vi "tcp_客户端_接收.vi"(0 "IP地址":string="127.0.0.1" caption="对方公网访问地址", 1 "端口号":i32=6314, 2 "储存路径":path=path "D:/AA") -> ()   [LabVIEW 2016, in "自动更新.lvlib" / "TCP文件传输系统.lvlib" / "TCP接收文件.lvlib"]
panel:
  out "运行中":bool
  out "单包大小":i32
  in  "分一包（兆）":i64=40
  out "已收百分比":string
  out "帧数":i32
  out "帧号":i32
  out "生成新的保存路径":path
  out "需接收次数":i32
  out "文件名":string
  out "已收次数":i32
  out "error out":errorcluster
  out "当前步骤":T1(ring)
  out "错误输出":errorcluster
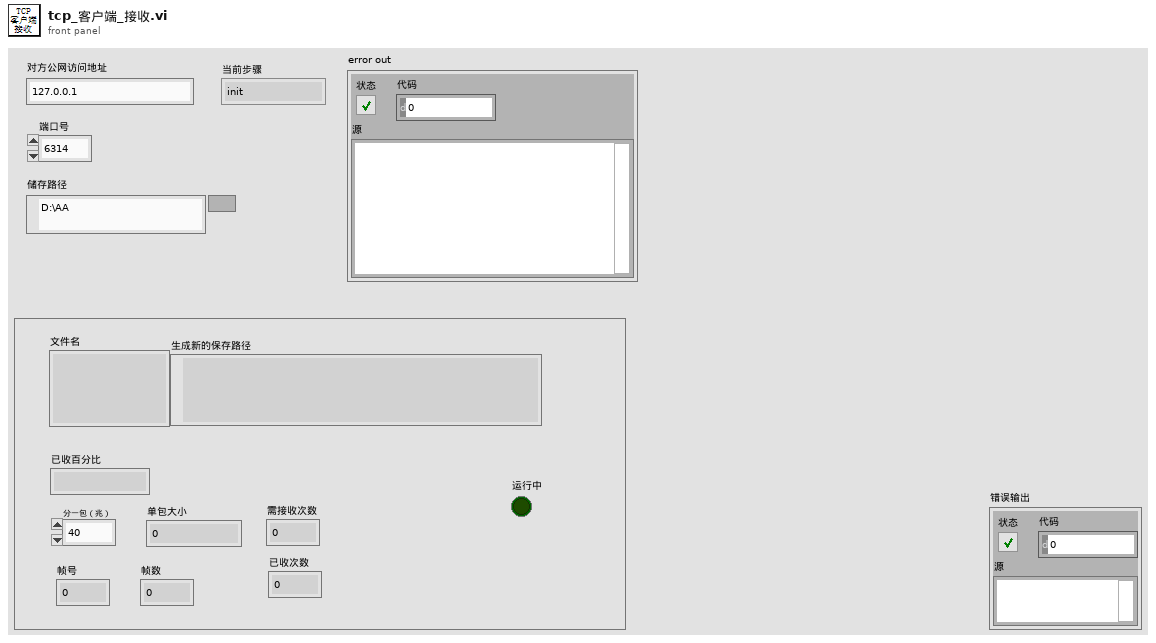
[diagram p1: front panel]
types:
  T1 = enum16{"init", "receivehead", "receivecontent", "receivesuccess", "over"}
  T2 = enum16{"open", "replace", "create", "open or create", "replace or create", "replace or create with confirmation"}
  T3 = cluster{"网络灯":bool, "接收中":bool, "已接收百分比":u8, "接收成功次数":dbl, "当前步骤":enum16{"init", "receivehead", "receivecontent", "receivesuccess", "over"}, "文件名":string, "error out":errorcluster}
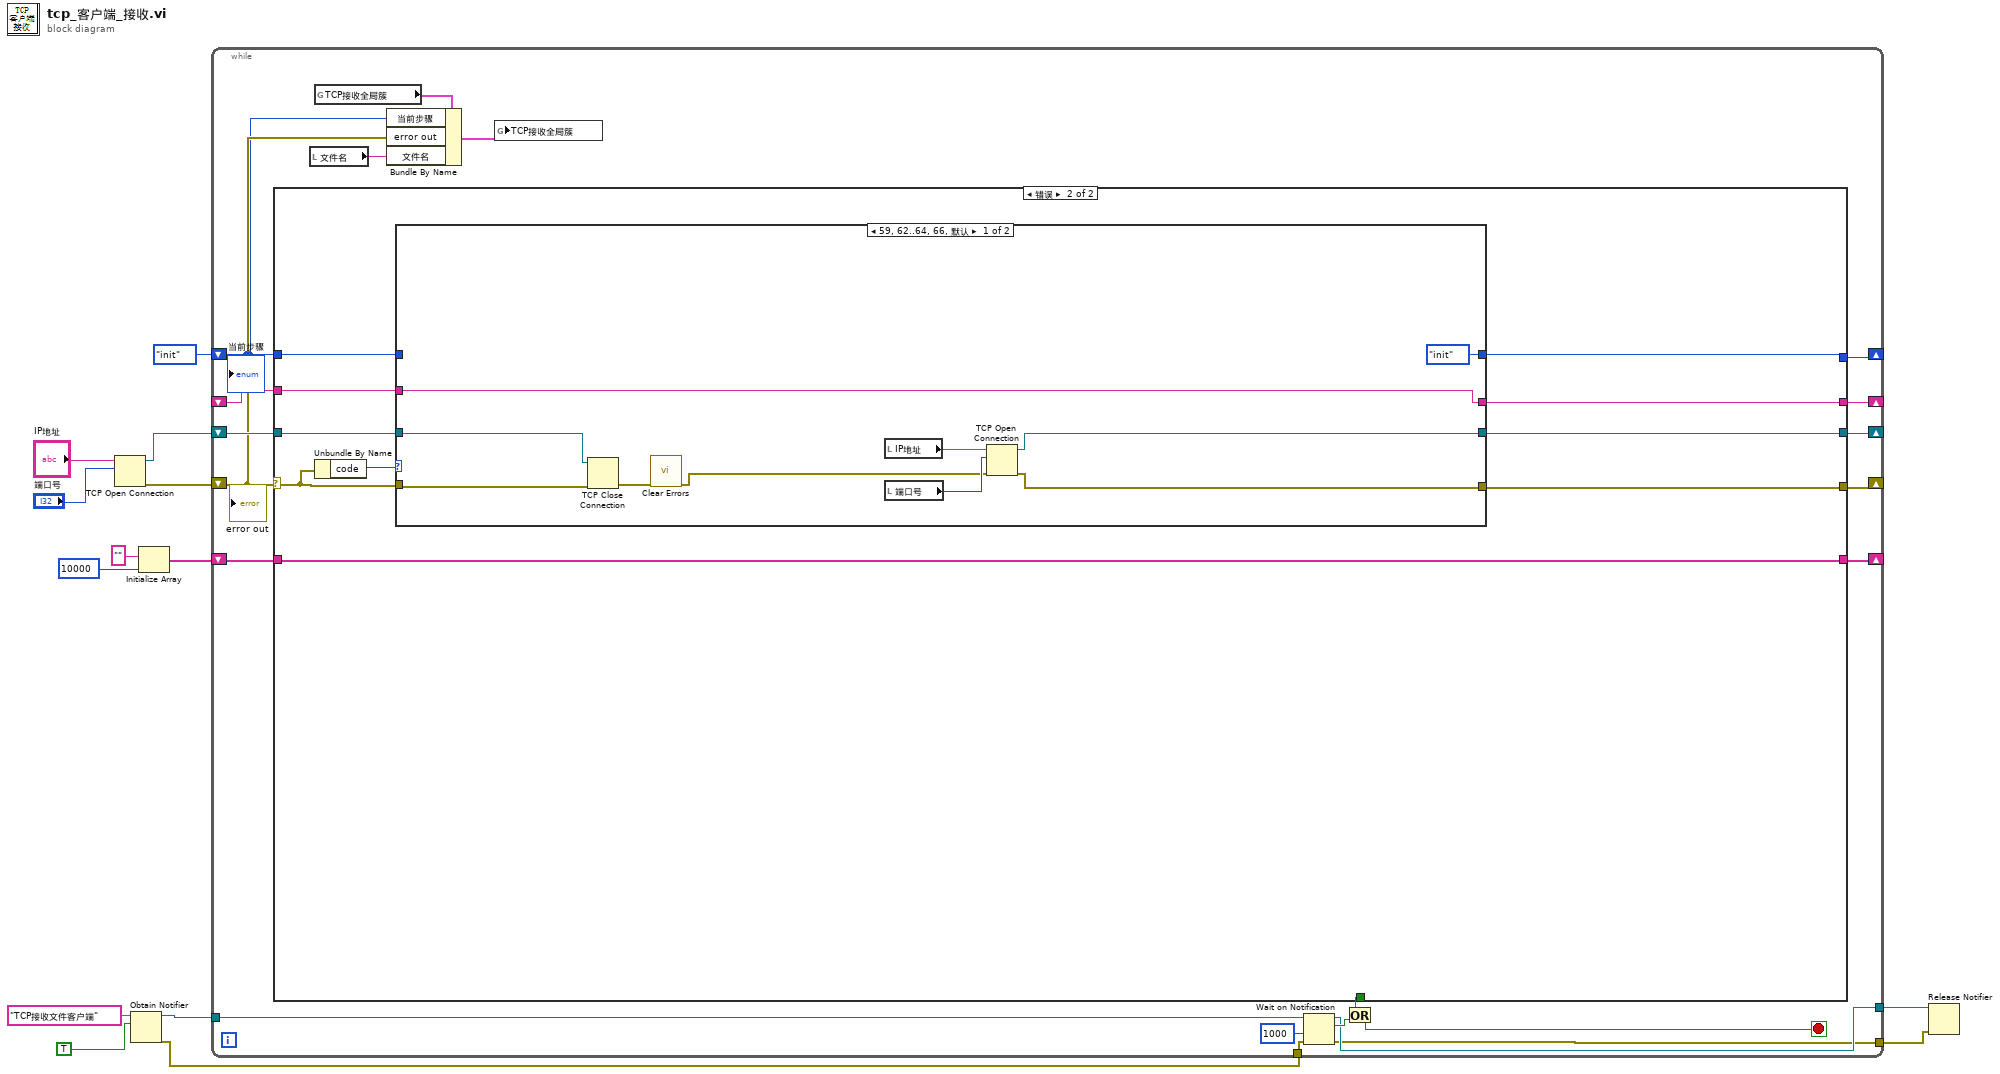
[diagram p0: block diagram]
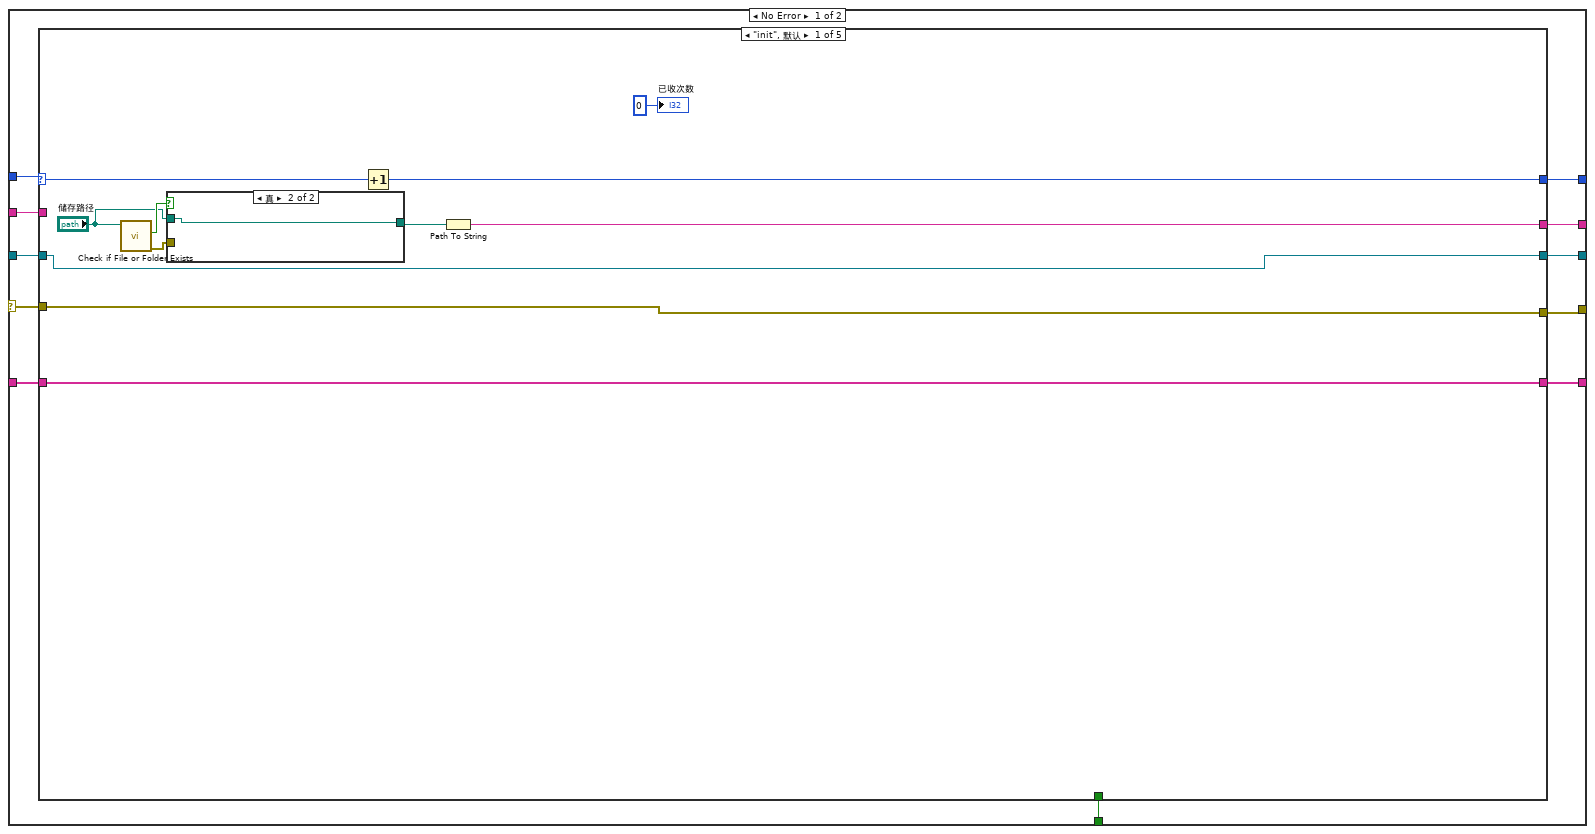
[diagram p2: hidden frame]
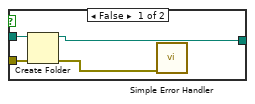
[diagram p3: hidden frame]
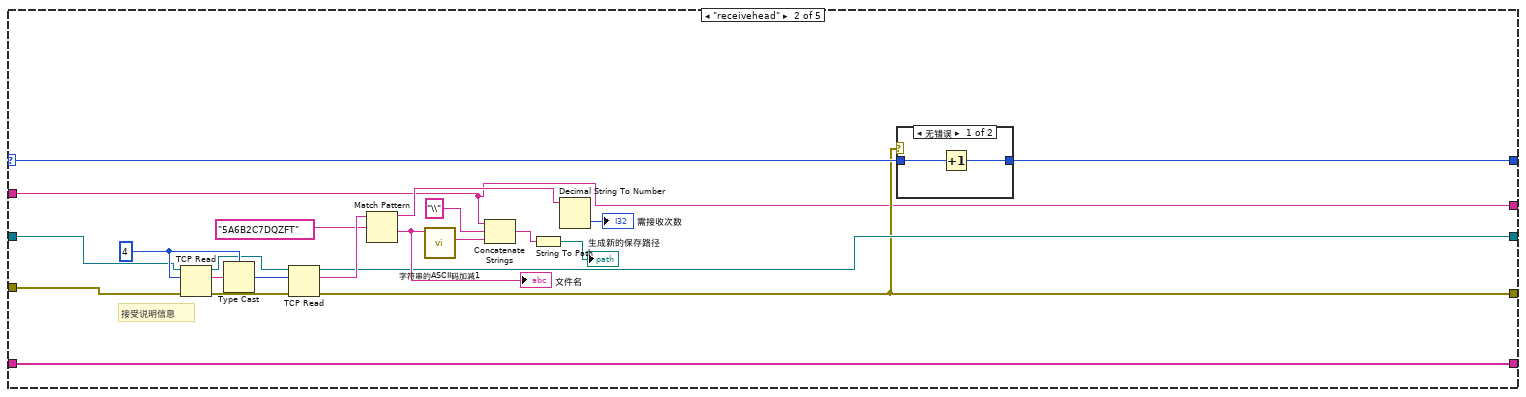
[diagram p4: hidden frame]
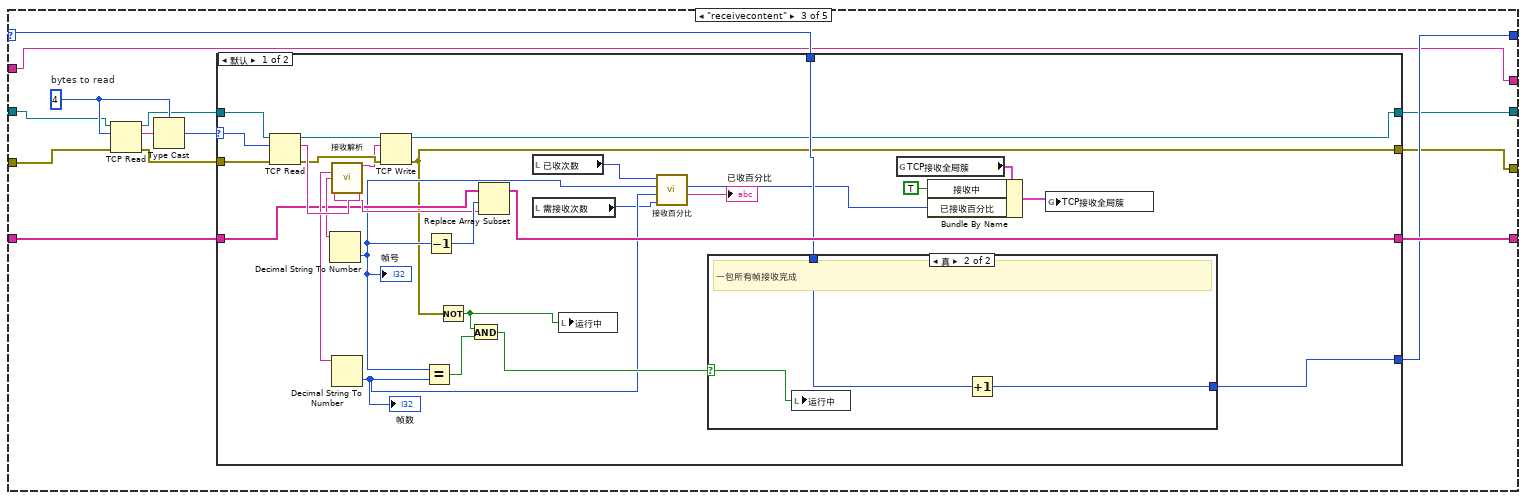
[diagram p6: hidden frame]
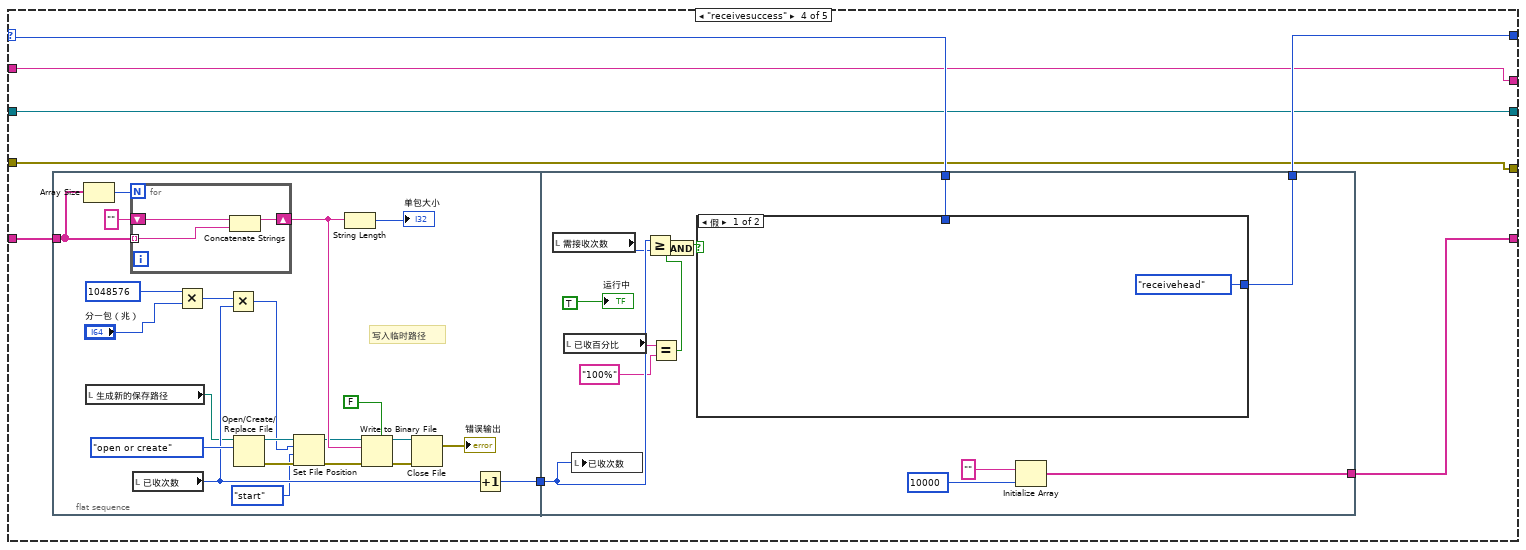
[diagram p9: hidden frame]
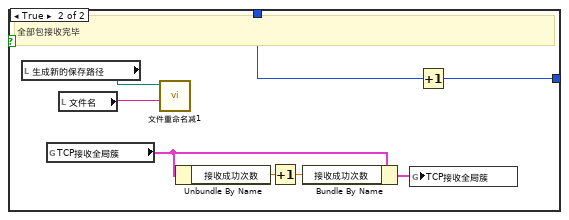
[diagram p10: hidden frame]
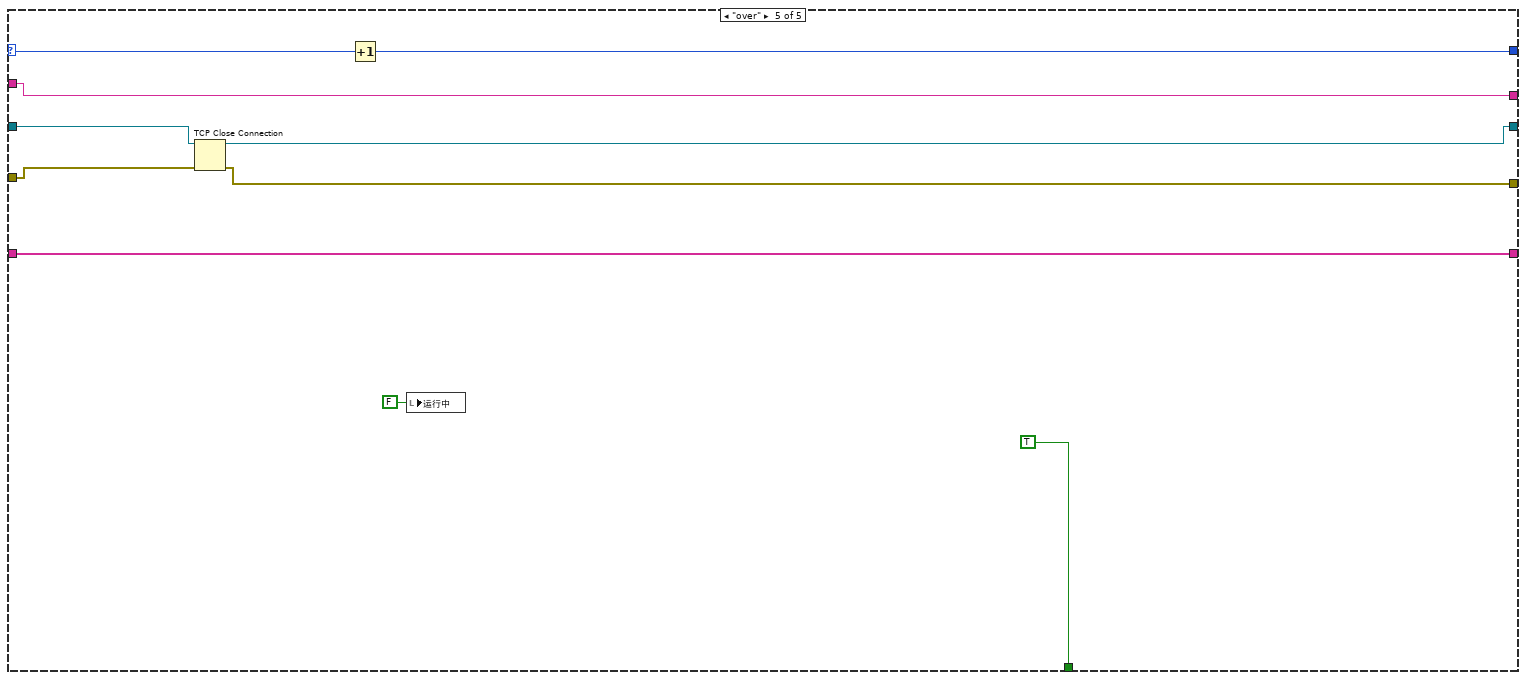
[diagram p11: hidden frame]
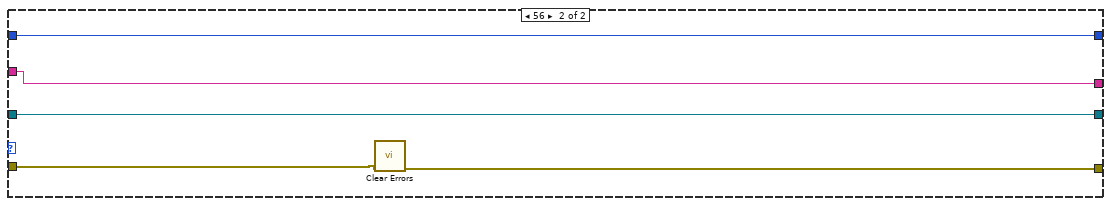
[diagram p12: hidden frame]
diagram:
  n1 = TCP Open Connection(address="IP地址", remote port or service name="端口号") -> (connection ID=w8:refnum<k5>, error out=w9:errorcluster)  [unwired: 3 in]
  n2 = Obtain Notifier(name (unnamed)="TCP接收文件客户端" ("名称（未命名）"), notification data type=TRUE) -> (notifier out=w6:refnum<notifier>, error out=w1:errorcluster)  [unwired: 2 in, 1 out]
  n3 = Initialize Array("", 10000 ("维数大小")) -> (w7:string[])
  n4 = while {
    shift-right: [w35] -> _
    shift-left: T1."init" -> [w16]
    shift-right: [w33] -> _
    shift-left: w9 -> [w17]
    shift-right: [w31] -> _
    shift-left: w8 -> [w32]
    shift-right: [w30] -> _
    shift-left: _ -> [w29]
    shift-right: [w27] -> _
    shift-left: w7 -> [w28]
    tunnel: w6 -> [w26]
    tunnel: [w22] -> w3
    tunnel: [w21] -> w2
    tunnel: w1 -> [w20]
    stop <- w25 stop-if-true
    n5 = case shown="错误" w17 {
      selector: w17 -> [w41 w212]
      tunnel: w16 -> [w46 w208]
      tunnel: [w45 w207] -> w35
      tunnel: [w44 _] -> w34
      tunnel: [w39 w211] -> w33
      tunnel: w32 -> [w42 w210]
      tunnel: [w38 w209] -> w31
      tunnel: [w43 w205] -> w30
      tunnel: w29 -> [w40 w206]
      tunnel: w28 -> [w37 w204]
      tunnel: [w36 w204] -> w27
      frame No Error {
        n6 = case shown="\"init\", 默认" w46 {
          selector: w46 -> [w57 w84 w92 w142 w203]
          tunnel: [w56 w83 w91 w143 w202] -> w45
          tunnel: [_ _ _ _ TRUE] -> w44
          tunnel: [w50 w64 w88 w139 w194] -> w43
          tunnel: w42 -> [w49 w75 w98 w140 w199]
          tunnel: w41 -> [w48 w74 w99 w141 w198]
          tunnel: w40 -> [_ w64 w88 w139 w194]
          tunnel: [w48 w65 w90 w141 w196] -> w39
          tunnel: [w49 w66 w89 w140 w197] -> w38
          tunnel: w37 -> [w47 w63 w96 w145 w195]
          tunnel: [w47 w63 w93 w144 w195] -> w36
          frame "init", Default {
            n7 = call <vilib>:"Check if File or Folder Exists.vi"("path"="储存路径") -> ("error out"=w53:errorcluster, "file or folder exists?"=w54:bool)  [unwired: 8 in, 1 out]
            n8 = case shown="真" w54 {
              tunnel: "储存路径" -> [w61 w62]
              tunnel: w53 -> [w60 _]
              tunnel: [w59 w62] -> w51
              frame False {
                n9 = Create Folder(path (use dialog)=w61, error in=w60) -> (created path=w59:path, error out=w58:errorcluster)  [unwired: 1 in, 1 out]
                n10 = call <vilib>:"Simple Error Handler.vi"("error in (no error)"=w58) -> ()  [unwired: 4 in, 5 out]
              }
              frame True {
              }
            }
            n11 = Increment(x=w57) -> (x+1=w56:T1)
            n12 = Path To String(path=w51) -> (string=w50:string)
            "已收次数" <- i64 0 ("已发次数")
          }
          frame "receivehead" {
            w82 = 4 ("读取的字节")
            # "接受说明信息"
            n13 = TCP Read(connection ID=w75, bytes to read=w82, error in (no error)=w74) -> (connection ID out=w78:refnum<k5>, data out=w81:string, error out=w79:errorcluster)  [unwired: 2 in]
            n14 = Type Cast(type=w82, x=w81) -> (*(type *) &x=w80:i32)
            n15 = TCP Read(connection ID=w78, bytes to read=w80, error in (no error)=w79) -> (connection ID out=w66:refnum<k5>, data out=w77:string, error out=w65:errorcluster)  [unwired: 2 in]
            n16 = Match Pattern(string=w77, regular expression="5A6B2C7DQZFT" ("正则表达式")) -> (before substring=w70:string, after substring=w73:string)  [unwired: 1 in, 2 out]
            "文件名" <- w73
            n17 = call "字符串的ASCII码加减1.vi"("原字符串"=w73) -> ("ASCII码"=w72:string)  [unwired: 10 in]
            n18 = Concatenate Strings(w64, "\\" ("字符串"), w72) -> (w67:string)
            n19 = String To Path(string=w67) -> (path=→"生成新的保存路径":path)
            n20 = Decimal String To Number(string=w70) -> (number=→"需接收次数":i32)  [unwired: 2 in, 1 out]
            n21 = case shown="无错误" w65 {
              tunnel: w84 -> [w86 w87]
              tunnel: [w85 w87] -> w83
              frame No Error {
                n22 = Increment(x=w86) -> (x+1=w85:T1)
              }
              frame Error {
              }
            }
          }
          frame "receivecontent" {
            w101 = 4  # bytes to read
            n23 = TCP Read(connection ID=w98, bytes to read=w101, error in (no error)=w99) -> (connection ID out=w95:refnum<k5>, data out=w100:string, error out=w94:errorcluster)  [unwired: 2 in]
            n24 = Type Cast(type=w101, x=w100) -> (*(type *) &x=w97:i32)
            n25 = case shown="默认" w97 {
              selector: w97 -> [w118 _]
              tunnel: w96 -> [w121 w137]
              tunnel: w95 -> [w120 w135]
              tunnel: w94 -> [w119 w136]
              tunnel: [w114 w137] -> w93
              tunnel: w92 -> [w112 w138]
              tunnel: [w111 w138] -> w91
              tunnel: [w110 w136] -> w90
              tunnel: [w109 w135] -> w89
              frame Default {
                n26 = TCP Read(connection ID=w120, bytes to read=w118, error in (no error)=w119) -> (connection ID out=w127:refnum<k5>, data out=w130:string, error out=w126:errorcluster)  [unwired: 2 in]
                n27 = call "接收解析.vi"("data in"=w130) -> ("重算CRC32"=w124:string, "帧数"=w125:string, "帧号"=w129:string, "帧内容"=w123:string)  [unwired: 3 in, 8 out]
                n28 = Decimal String To Number(string=w129) -> (number=w116:i32)  [unwired: 2 in, 1 out]
                "帧号" <- w116
                n29 = Decimal String To Number(string=w125) -> (number=w103:i32)  [unwired: 2 in, 1 out]
                "帧数" <- w103
                n30 = TCP Write(connection ID=w127, data in=w124, error in (no error)=w126) -> (connection ID out=w109:refnum<k5>, error out=w110:errorcluster)  [unwired: 1 in, 1 out]
                n31 = Equal?(x=w116, y=w103) -> (x = y?=w122:bool)
                n32 = Decrement(x=w116) -> (x-1=w128:i32)
                n33 = Not(x=w110) -> (.not. x?=w108:bool)
                n34 = And(x=w108, y=w122) -> (x .and. y?=w113:bool)
                n35 = Replace Array Subset(array=w121, new element=w123, index=w128) -> (w114:string[])
                n36 = local read "已收次数"() -> (w117:i32)
                n37 = local read "需接收次数"() -> (w102:i32)
                n38 = local write "运行中"(w108) -> ()
                n39 = call "接收百分比.vi"("需发送次数"=w102, "帧数"=w103, "帧号"=w116, "已收次数"=w117) -> (1:"已收百分比"=→"已收百分比":string, 2:"已收百分比"=w104:u8)  [unwired: 6 in]
                n40 = case shown="真" w113 {
                  selector: w113 -> [_ w132]
                  tunnel: w112 -> [w131 w134]
                  tunnel: [w131 w133] -> w111
                  frame False {
                    # "重复接收"
                  }
                  frame True {
                    # "一包所有帧接收完成"
                    n41 = local write "运行中"(w132) -> ()
                    n42 = Increment(x=w134) -> (x+1=w133:T1)
                  }
                }
                n43 = global read "全局变量1.vi" "TCP接收全局簇"() -> (w105:T3)
                n44 = Bundle By Name(cluster=w105, "接收中"=TRUE, "已接收百分比"=w104) -> (w106:T3)
                n45 = global write "全局变量1.vi" "TCP接收全局簇"(w106) -> ()
              }
              frame ..0 {
                # "content为空"
              }
            }
          }
          frame "receivesuccess" {
            n46 = flat-sequence {
              tunnel: w145 -> [w160]
              tunnel: [w168] -> w146
              tunnel: w146 -> [w178]
              tunnel: [w182] -> w144
              tunnel: w142 -> [w180]
              tunnel: [w179] -> w143
              frame #0 {
                # "写入临时路径"
                n47 = Array Size(array=w160) -> (size(s)=w161:i32)
                n48 = local read "生成新的保存路径"() -> (w147:path)
                n49 = for {
                  N: w161 -> [_]
                  shift-right: [w171] -> w159
                  shift-left: "" -> [w170]
                  tunnel: w160 -> [w169] mode=indexing
                  n50 = Concatenate Strings(w170, w169) -> (w171:string)
                }
                n51 = local read "已收次数"() -> (w153:i32)
                n52 = Multiply(x=i64 1048576, y="分一包（兆）") -> (x*y=w149:i64)
                n53 = Multiply(x=w149, y=w153) -> (x*y=w152:i64)
                n54 = Open/Create/Replace File(file path (use dialog)=w147, operation (0:open)=T2."open or create" ("操作(0:open)")) -> (refnum out=w156:refnum<file>, error out=w157:errorcluster)  [unwired: 4 in, 1 out]
                n55 = Set File Position(offset (in bytes) (0)=w152, refnum=w156, from (0:start)=enum16{"start", "end", "current"}."start" ("自（0:起始）"), error in=w157) -> (refnum out=w154:refnum<file>, error out=w155:errorcluster)
                n56 = String Length(string=w159) -> (length=→"单包大小":i32)
                n57 = Write to Binary File(file (use dialog)=w154, data=w159, error in=w155, 5:FALSE ("预置数组或字符串大小？(T)")) -> (refnum out=w166:refnum<file>, error out=w167:errorcluster)  [unwired: 2 in, 1 out]
                n58 = Close File(refnum=w166, error in=w167) -> (error out=→"错误输出":errorcluster)  [unwired: 1 out]
                n59 = Increment(x=w153) -> (x+1=w168:i32)
              }
              frame #1 {
                n60 = local read "需接收次数"() -> (w177:i32)
                n61 = local read "已收百分比"() -> (w175:string)
                n62 = local write "已收次数"(w178) -> ()
                n63 = Greater Or Equal?(x=w178, y=w177) -> (x >= y?=w176:bool)
                n64 = Equal?(x=w175, y="100%" ("已收百分比")) -> (x = y?=w172:bool)
                n65 = And(x=w176, y=w172) -> (x .and. y?=w173:bool)
                n66 = case shown="假" w173 {
                  tunnel: w180 -> [_ w187]
                  tunnel: [T1."receivehead" w186] -> w179
                  frame False {
                  }
                  frame True {
                    # "全部包接收完毕"
                    n67 = local read "生成新的保存路径"() -> (w193:path)
                    n68 = global read "全局变量1.vi" "TCP接收全局簇"() -> (w188:T3)
                    n69 = local read "文件名"() -> (w192:string)
                    n70 = call "文件重命名减1.vi"("名称或相对路径"=w192, "源路径"=w193) -> ()  [unwired: 10 in]
                    n71 = Unbundle By Name(w188) -> ("接收成功次数"=w189:dbl)
                    n72 = Increment(x=w189) -> (x+1=w190:dbl)
                    n73 = Bundle By Name(cluster=w188, "接收成功次数"=w190) -> (w191:T3)
                    n74 = global write "全局变量1.vi" "TCP接收全局簇"(w191) -> ()
                    n75 = Increment(x=w187) -> (x+1=w186:T1)
                  }
                }
                n76 = Initialize Array("", 10000 ("维数大小")) -> (w182:string[])
                "运行中" <- TRUE ("运行指示灯")
              }
            }
          }
          frame "over" {
            n77 = TCP Close Connection(connection ID=w199, error in (no error)=w198) -> (connection ID out=w197:refnum<k5>, error out=w196:errorcluster)  [unwired: 1 in]
            n78 = Increment(x=w203) -> (x+1=w202:T1)
            n79 = local write "运行中"(FALSE ("运行中")) -> ()
          }
        }
      }
      frame Error {
        n80 = Unbundle By Name(w212) -> ("code"=w213:i32)
        n81 = case shown="59, 62..64, 66, 默认" w213 {
          tunnel: w212 -> [w220 w228]
          tunnel: [w216 w227] -> w211
          tunnel: w210 -> [w219 w224]
          tunnel: [w217 w224] -> w209
          tunnel: w208 -> [_ w226]
          tunnel: [T1."init" w226] -> w207
          tunnel: w206 -> [w215 w225]
          tunnel: [w215 w225] -> w205
          frame 59, 62..64, 66, Default {
            n82 = TCP Close Connection(connection ID=w219, error in (no error)=w220) -> (error out=w221:errorcluster)  [unwired: 1 in, 1 out]
            n83 = call <vilib>:"Clear Errors.vi"("error in (no error)"=w221) -> ("error out"=w218:errorcluster)  [unwired: 5 in, 1 out]
            n84 = local read "IP地址"() -> (w223:string)
            n85 = local read "端口号"() -> (w222:i32)
            n86 = TCP Open Connection(address=w223, remote port or service name=w222, error in (no error)=w218) -> (connection ID=w217:refnum<k5>, error out=w216:errorcluster)  [unwired: 2 in]
          }
          frame 56 {
            n87 = call <vilib>:"Clear Errors.vi"("error in (no error)"=w228) -> ("error out"=w227:errorcluster)  [unwired: 5 in, 1 out]
          }
        }
      }
    }
    n88 = local read "文件名"() -> (w15:string)
    n89 = global read "全局变量1.vi" "TCP接收全局簇"() -> (w18:T3)
    n90 = Bundle By Name(cluster=w18, "当前步骤"=w16, "error out"=w17, "文件名"=w15) -> (w19:T3)
    n91 = global write "全局变量1.vi" "TCP接收全局簇"(w19) -> ()
    n92 = Wait on Notification(notifier=w26, timeout in ms (-1)=1000 ("超时毫秒(-1)"), error in (no error)=w20) -> (notifier out=w22:refnum<notifier>, notification=w24:bool, error out=w21:errorcluster)  [unwired: 1 in, 1 out]
    n93 = Or(x=w34, y=w24) -> (x .or. y?=w25:bool)
    "当前步骤" <- w16
    "error out" <- w17
  }
  n94 = Release Notifier(notifier=w3, error in (no error)=w2) -> ()  [unwired: 1 in, 3 out]
